vi "Main.vi"() -> ()   [LabVIEW 2013, in "Simple Sequence Editor.lvlib"]
uses:
  Simple Sequence Editor.lvlib
  Types/UI.PropertiesTypes.ctl
  Types/StateVariables.ctl
  Types/ChannelProperties.ctl
  <vilib>/Utility/miscctls.llb/LVBoundsTypeDef.ctl
panel:
  in  "Sequence":i32[](listbox)
  in  "View":T1=enum."Sequence Properties"
  in  "Abort Channel":string(combo)
  in  "Step Information Channel":string(combo)
  out "Graph":waveform(dbl)[](graph)
  out "Path":path
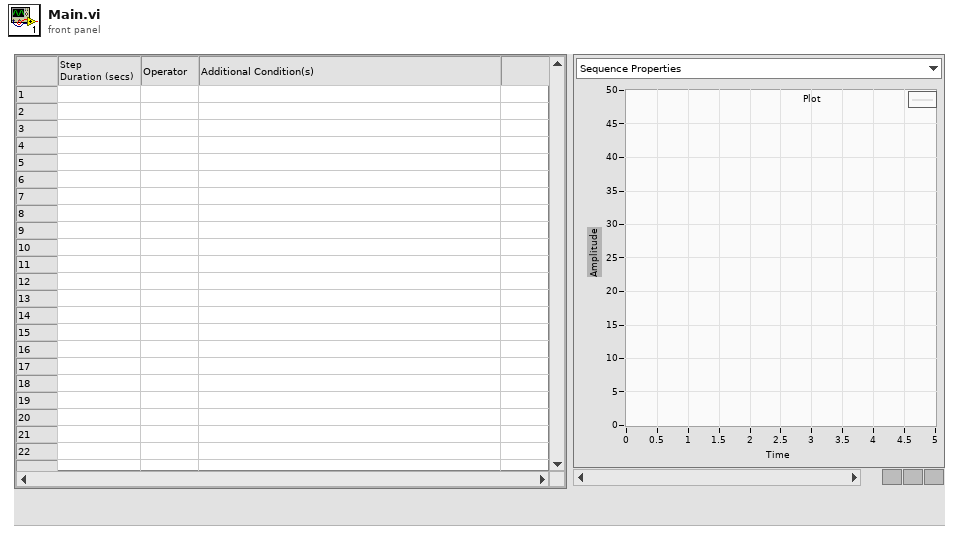
[diagram p1: front panel]
types:
  T1 = typedef "Simple Sequence Editor.lvlib/UI.PropertiesTypes.ctl" = enum8{"Step Properties", "Sequence Properties"}
  T2 = typedef "Simple Sequence Editor.lvlib/StateVariables.ctl" = cluster{"Aliases.All":T3[], "Aliases.Outputs":T3[], "UI.Sequence#ofColumns":i32, "SysDef.Path":path, "UI.SequenceRef":refnum<vi>, "UI.StepInformationRef":refnum<vi>, "UI.AbortRef":refnum<vi>, "UI.GraphRef":refnum<vi>, "UI.ViewRef":refnum<vi>}
  T3 = typedef "Simple Sequence Editor.lvlib/ChannelProperties.ctl" = cluster{"Name":string, "NodePath":string, "ScaleUnits":string}
  T4 = typedef "LVBoundsTypeDef.ctl" = cluster{"Width":u32, "Height":u32}
  T5 = enum16{"open", "replace", "create", "open or create", "replace or create", "replace or create with confirmation"}
  T6 = typedef "LVPoint32TypeDef.ctl" = cluster{"Horizontal":i32, "Vertical":i32}
  T7 = typedef "Simple Sequence Editor.lvlib/Compiled.RTSequenceProperties.ctl" = cluster{"Channels":T3[], "Steps":T8[]}
  T8 = typedef "Simple Sequence Editor.lvlib/Compiled.StepProperties.ctl" = cluster{"IOState":T9, "Condition":T12}
  T9 = typedef "Simple Sequence Editor.lvlib/Compiled.IOStateProperties.ctl" = cluster{"Duration":dbl, "Elements":T10[]}
  T10 = typedef "Simple Sequence Editor.lvlib/Compiled.StepElementProperties.ctl" = cluster{"Channel":T3, "Step":T11, "Parameters":dbl[]}
  T11 = typedef "Simple Sequence Editor.lvlib/StepTypes.ctl" = enum8{"Step", "iStep", "Ramp", "Unchanged", "Unknown"}
  T12 = typedef "Simple Sequence Editor.lvlib/Compiled.StepCondition.ctl" = cluster{"First Opreation":T13, "Expression":string}
  T13 = typedef "Simple Sequence Editor.lvlib/OperationTypes.ctl" = enum8{"None", "&&", "||"}
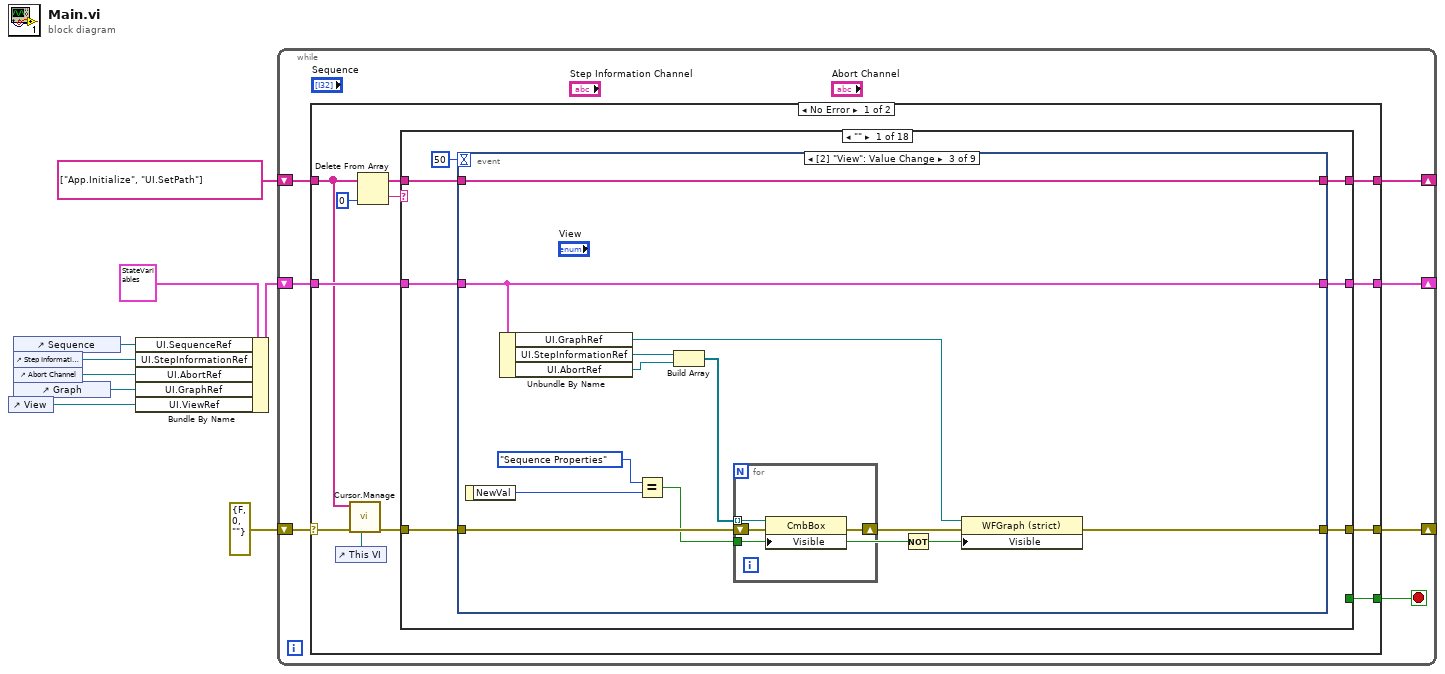
[diagram p0: block diagram]
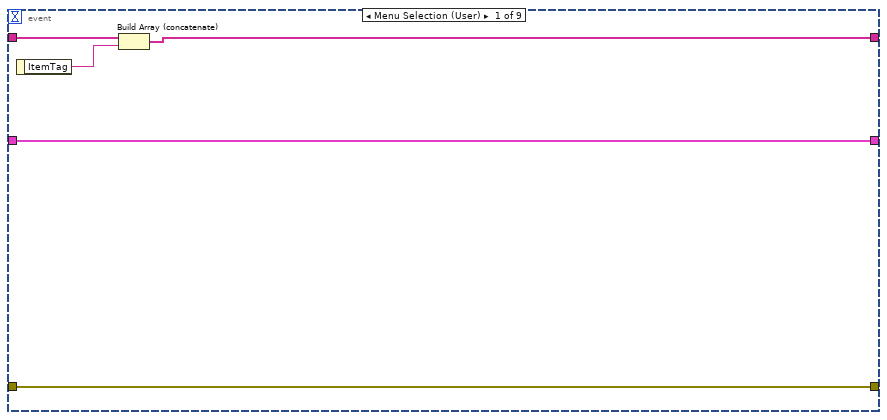
[diagram p2: hidden frame]
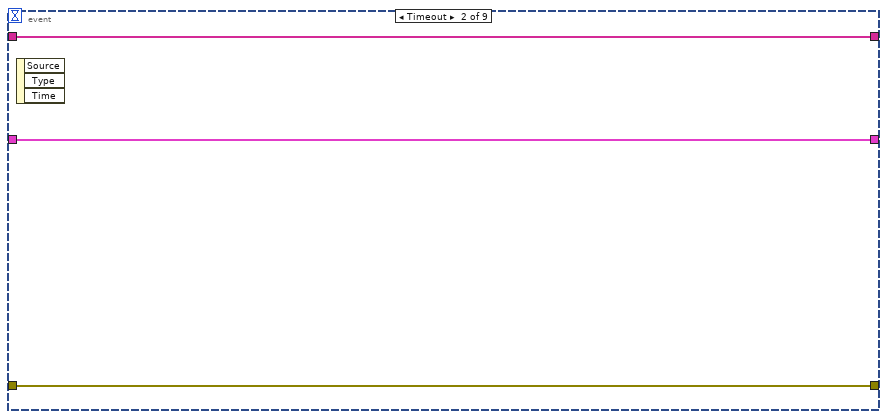
[diagram p3: hidden frame]
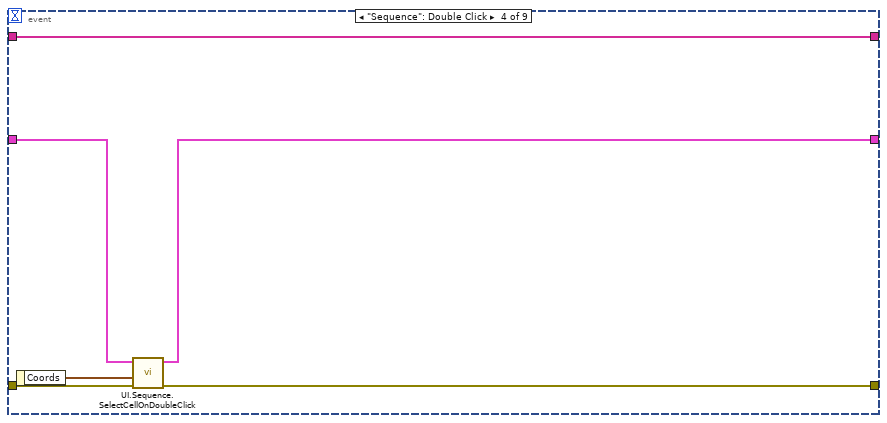
[diagram p4: hidden frame]
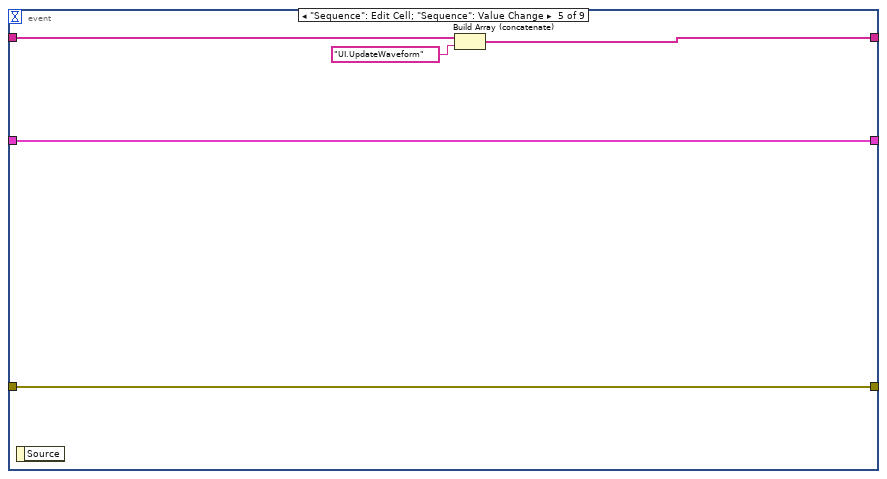
[diagram p5: hidden frame]
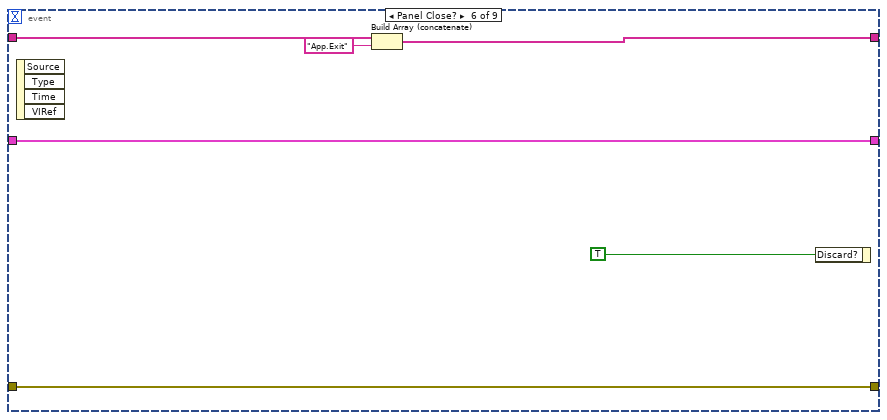
[diagram p6: hidden frame]
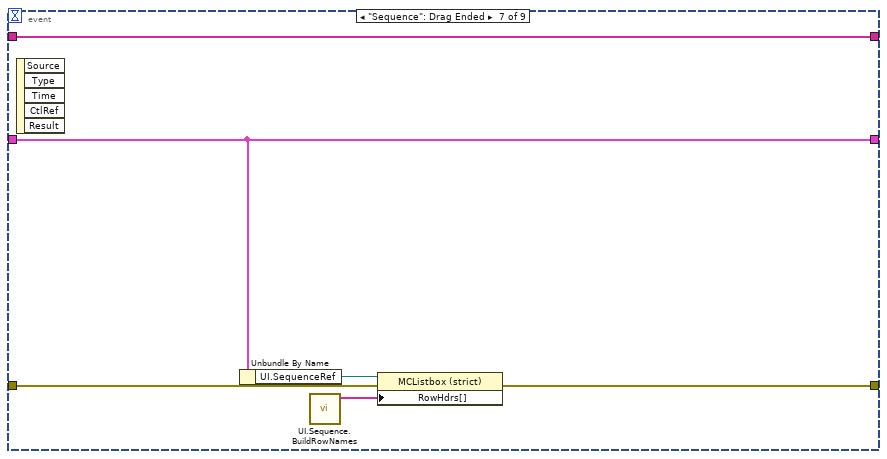
[diagram p7: hidden frame]
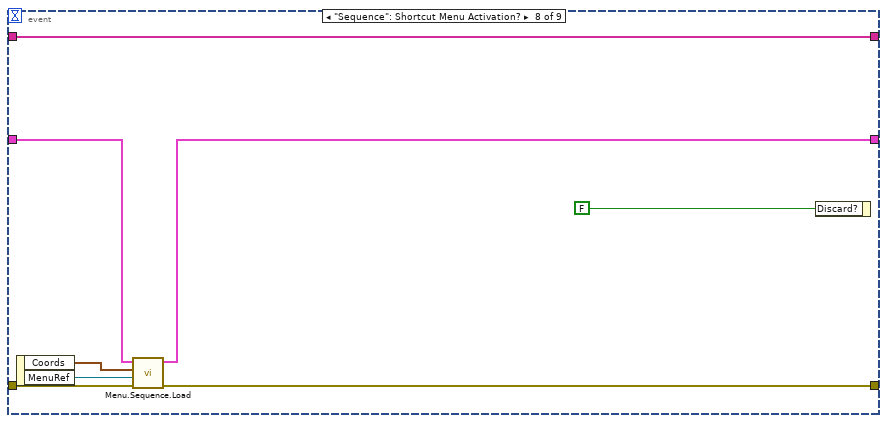
[diagram p8: hidden frame]
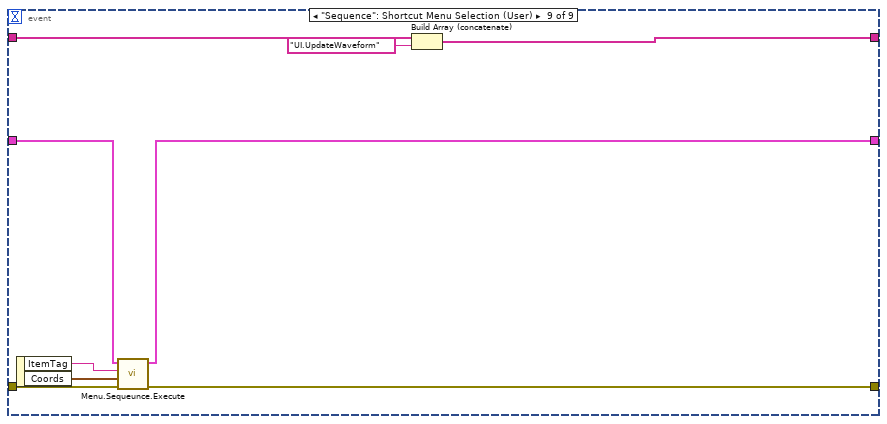
[diagram p9: hidden frame]
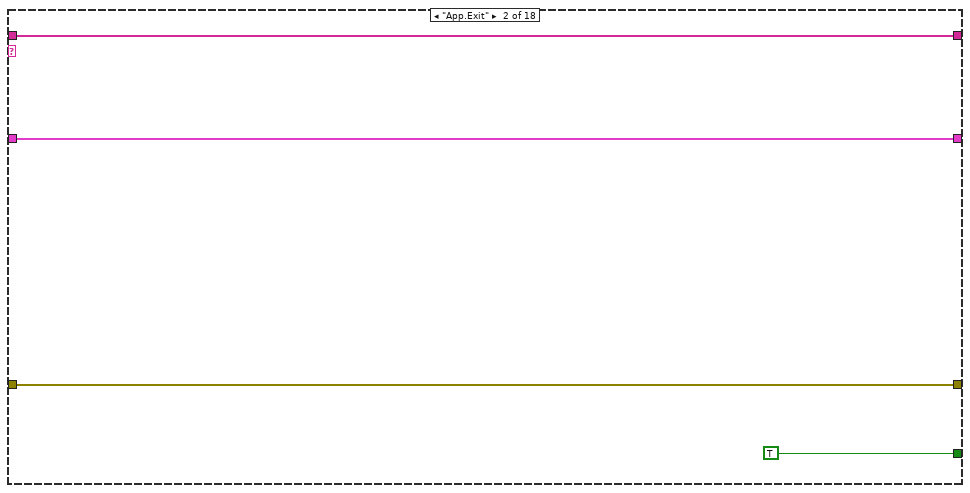
[diagram p10: hidden frame]
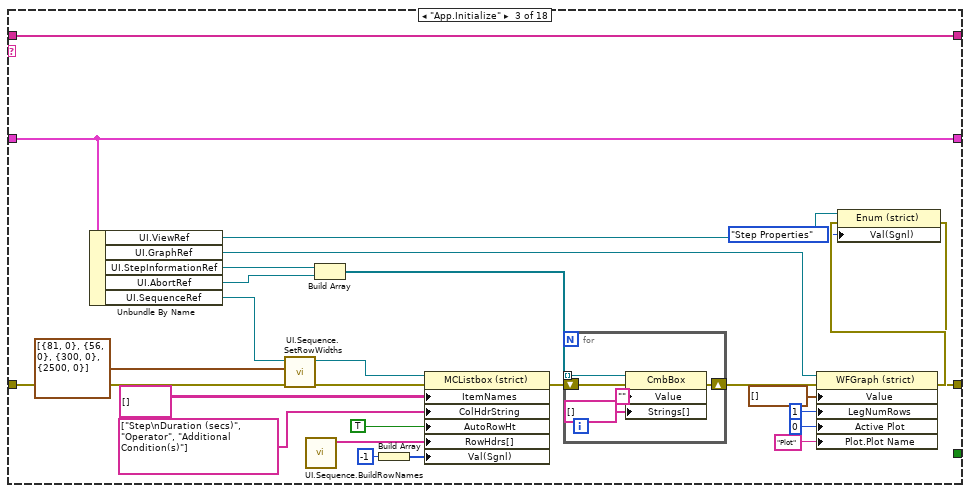
[diagram p11: hidden frame]
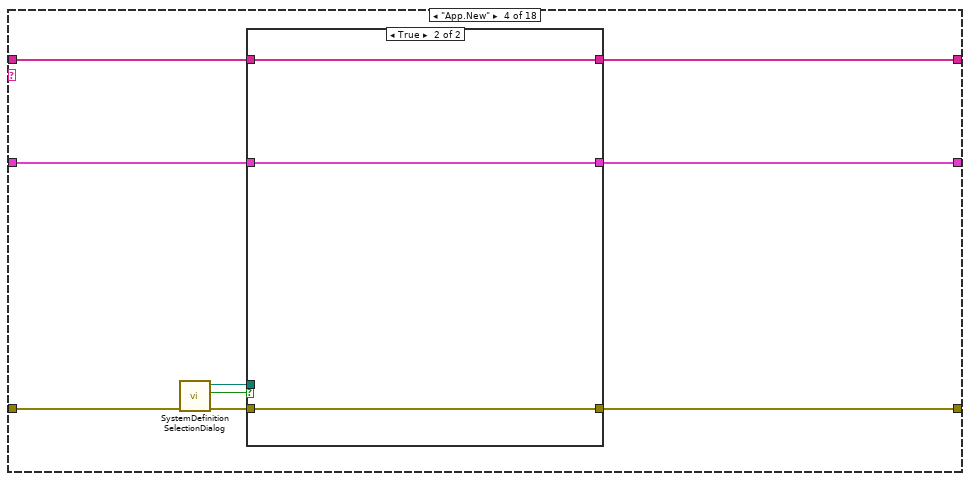
[diagram p12: hidden frame]
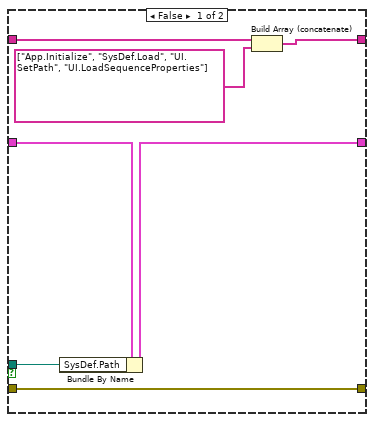
[diagram p13: hidden frame]
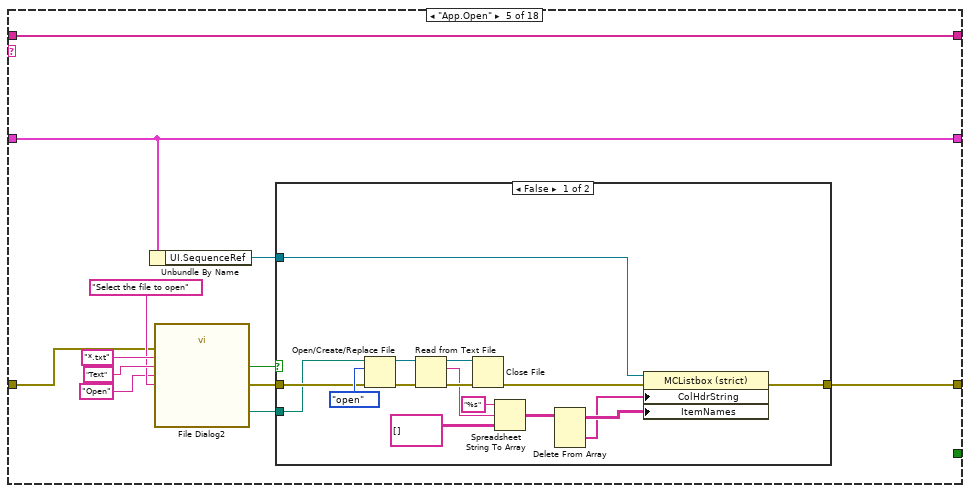
[diagram p14: hidden frame]
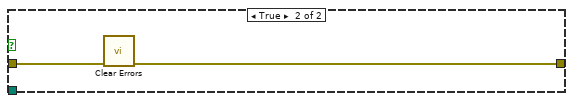
[diagram p15: hidden frame]
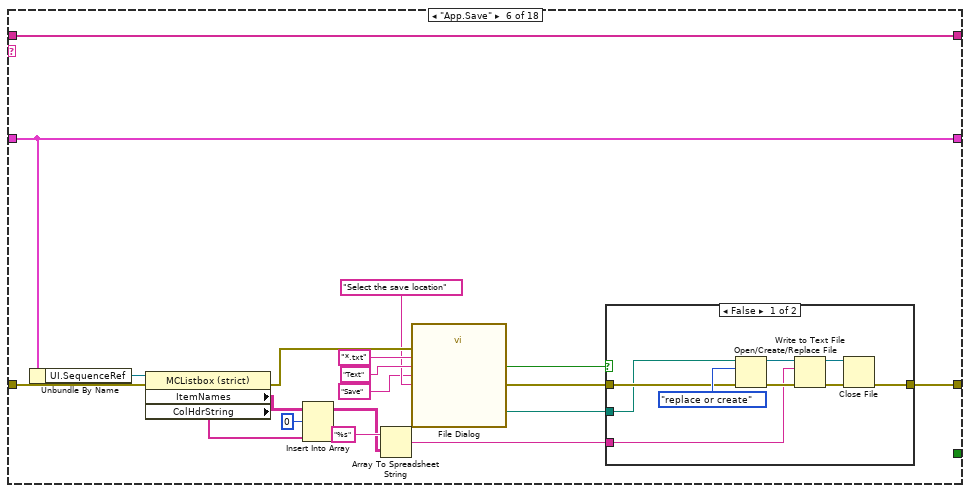
[diagram p16: hidden frame]
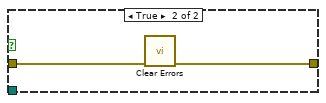
[diagram p17: hidden frame]
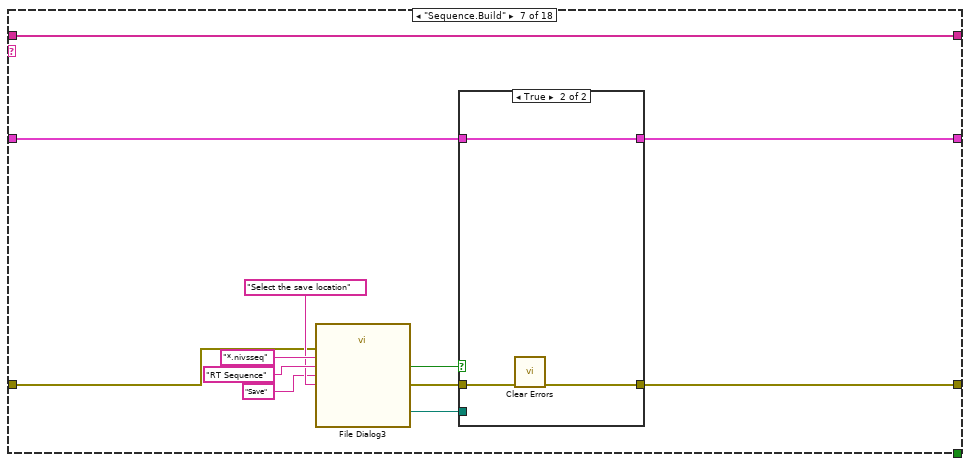
[diagram p18: hidden frame]
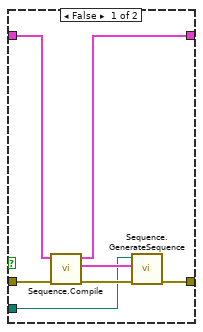
[diagram p19: hidden frame]
diagram:
  n1 = control-ref of="View"() -> (w1:refnum<vi>)
  n2 = control-ref of="Sequence"() -> (w5:refnum<vi>)
  n3 = control-ref of="Step Information Channel"() -> (w4:refnum<vi>)
  n4 = control-ref of="Abort Channel"() -> (w3:refnum<vi>)
  n5 = control-ref of="Graph"() -> (w2:refnum<vi>)
  n6 = Bundle By Name(cluster=T2 {"Aliases.All"=[], "Aliases.Outputs"=[], "UI.Sequence#ofColumns"=0, "SysDef.Path"=path "", "UI.SequenceRef"=refnum, "UI.StepInformationRef"=refnum, "UI.AbortRef"=refnum, "UI.GraphRef"=refnum, "UI.ViewRef"=refnum}, "UI.SequenceRef"=w5, "UI.StepInformationRef"=w4, "UI.AbortRef"=w3, "UI.GraphRef"=w2, "UI.ViewRef"=w1) -> (w6:T2)
  n7 = while {
    shift-right: [w15] -> _
    shift-left: string[] ["App.Initialize", "UI.SetPath"] -> [w16]
    shift-right: [w13] -> _
    shift-left: w6 -> [w14]
    shift-right: [w11] -> _
    shift-left: errorcluster {"status"=FALSE, "code"=0, "source"=""} ("error constant") -> [w12]
    stop <- w10 stop-if-true
    n8 = case shown="No Error" w12 {
      selector: w12 -> [w20 w326]
      tunnel: w16 -> [w21 w329]
      tunnel: [w27 w329] -> w15
      tunnel: w14 -> [w25 w328]
      tunnel: [w24 w328] -> w13
      tunnel: [w23 w325] -> w11
      tunnel: [w22 _] -> w10
      frame No Error {
        n9 = control-ref of="This VI"() -> (w17:refnum<vi>)
        n10 = call "Cursor.Manage.vi"("VI reference (current VI)"=w17, "error in (no error)"=w20, "Cmd list"=w21) -> ("error out"=w19:errorcluster)  [unwired: 8 in]
        n11 = Delete From Array(array=w21, index=0) -> (deleted portion=w28:string, array with subset deleted=w26:string[])  [unwired: 1 in]
        n12 = case shown="\"\"" w28 {
          tunnel: [w32 w104 w131 w137 w167 w204 w227 w240 w244 w250 w266 w267 w289 w294 w298 w312 w321 w324] -> w27
          tunnel: w26 -> [w31 w104 w131 w138 w167 w204 w227 w240 w244 w250 w266 w268 w290 w294 w298 w312 w321 w324]
          tunnel: w25 -> [w34 w103 w130 w141 w157 w203 w217 w239 w243 w249 w263 w271 w286 w291 w296 w307 w320 w323]
          tunnel: [w35 w103 w130 w139 w157 w203 w216 w239 w243 w249 w262 w269 w286 w291 w296 w308 w320 w323] -> w24
          tunnel: [w29 w102 w107 w142 w158 w199 w226 w238 w241 w247 w264 w272 w287 w292 w297 w309 w313 w322] -> w23
          tunnel: w19 -> [w30 w102 w125 w144 w159 w201 w221 w238 w242 w248 w259 w274 w287 w293 w297 w305 w314 w322]
          tunnel: [_ TRUE _ _ _ _ _ _ _ _ _ _ _ _ _ _ _ _] -> w22
          frame "" {
            n13 = event shown="[2] \"View\": Value Change" {
              selector: _ -> [_ _ _ _ _ _ _ _ _]
              dyn-events: _ -> [_ _ _ _ _ _ _ _ _]
              timeout: 50 -> [_ _ _ _ _ _ _ _ _]
              tunnel: [w37 w43 w56 w66 w68 w73 w83 w91 w93] -> w32
              tunnel: w31 -> [w39 w43 w56 w66 w71 w77 w83 w91 w100]
              tunnel: [w40 w42 w55 w61 w70 w76 w79 w87 w94] -> w35
              tunnel: w34 -> [w40 w42 w55 w62 w70 w76 w79 w84 w95]
              tunnel: [w38 w41 w47 w63 w69 w75 w80 w88 w96] -> w29
              tunnel: w30 -> [w38 w41 w51 w64 w69 w75 w81 w89 w97]
              event Menu Selection (User) {
                n14 = event-data() -> ("ItemTag"=w36:string)  [unwired: 1 in]
                n15 = Build Array (concatenate)(w39, w36) -> (w37:string[])
              }
              event Timeout {
                n16 = event-data() -> ()  [unwired: 1 in, 3 out]
              }
              event Value Change {
                n17 = event-data() -> ("NewVal"=w49:T1)  [unwired: 1 in]
                n18 = Unbundle By Name(w55) -> ("UI.GraphRef"=w46:refnum<vi>, "UI.StepInformationRef"=w54:refnum<vi>, "UI.AbortRef"=w53:refnum<vi>)
                n19 = Equal?(x=UI.PropertiesTypes."Sequence Properties" ("View"), y=w49) -> (x = y?=w45:bool)
                n20 = Build Array(w54, w53) -> (w52:refnum<vi>[])
                n21 = for {
                  tunnel: w52 -> [w60] mode=indexing
                  shift-right: [w58] -> w48
                  shift-left: w51 -> [w59]
                  tunnel: w45 -> [w57]
                  n22 = property class="CmbBox"(reference=w60, error in=w59, "Visible"=w57) -> (error out=w58:errorcluster)  [unwired: 1 out]
                }
                n23 = Not(x=w45) -> (.not. x?=w44:bool)
                n24 = property class="WFGraph (strict)"(reference=w46, error in=w48, "Visible"=w44) -> (error out=w47:errorcluster)  [unwired: 1 out]
              }
              event "Sequence": Double Click {
                n25 = event-data() -> ("Coords"=w65:T6)  [unwired: 1 in]
                n26 = call "UI.Sequence.SelectCellOnDoubleClick.vi"("error in (no error)"=w64, "Coords"=w65, "Cluster"=w62) -> ("error out"=w63:errorcluster, "Cluster out"=w61:T2)  [unwired: 7 in]
              }
              event "Sequence": Edit Cell; "Sequence": Value Change {
                n27 = event-data() -> ()  [unwired: 1 in, 1 out]
                n28 = Build Array (concatenate)(w71, "UI.UpdateWaveform" ("message")) -> (w68:string[])
              }
              event Panel Close? {
                n29 = event-data() -> ()  [unwired: 1 in, 4 out]
                n30 = Build Array (concatenate)(w77, "App.Exit") -> (w73:string[])
                n31 = event-data("Discard?"=TRUE) -> ()  [unwired: 1 in, 1 out]
              }
              event "Sequence": Drag Ended {
                n32 = event-data() -> ()  [unwired: 1 in, 5 out]
                n33 = Unbundle By Name(w79) -> ("UI.SequenceRef"=w78:refnum<vi>)
                n34 = call "UI.Sequence.BuildRowNames.vi"() -> ("Array"=w82:string[])  [unwired: 11 in]
                n35 = property class="MCListbox (strict)"(reference=w78, error in=w81, "RowHdrs[]"=w82) -> (error out=w80:errorcluster)  [unwired: 1 out]
              }
              event "Sequence": Shortcut Menu Activation? {
                n36 = event-data() -> ("Coords"=w85:T6, "MenuRef"=w86:refnum<k9>)  [unwired: 1 in]
                n37 = call "Menu.Sequence.Load.vi"("error in (no error)"=w89, "MenuRef"=w86, "Coords"=w85, "Cluster in"=w84) -> ("error out"=w88:errorcluster, "Cluster out"=w87:T2)  [unwired: 6 in]
                n38 = event-data("Discard?"=FALSE) -> ()  [unwired: 1 in, 1 out]
              }
              event "Sequence": Shortcut Menu Selection (User) {
                n39 = event-data() -> ("ItemTag"=w99:string, "Coords"=w98:T6)  [unwired: 1 in]
                n40 = call "Menu.Sequeunce.Execute.vi"("error in (no error)"=w97, "Coords"=w98, "ItemPath"=w99, "Cluster in"=w95) -> ("error out"=w96:errorcluster, "Cluster out"=w94:T2)  [unwired: 6 in]
                n41 = Build Array (concatenate)(w100, "UI.UpdateWaveform" ("message")) -> (w93:string[])
              }
            }
          }
          frame "App.Exit" {
          }
          frame "App.Initialize" {
            n42 = Unbundle By Name(w130) -> ("UI.ViewRef"=w109:refnum<vi>, "UI.GraphRef"=w115:refnum<vi>, "UI.StepInformationRef"=w117:refnum<vi>, "UI.AbortRef"=w118:refnum<vi>, "UI.SequenceRef"=w123:refnum<vi>)
            n43 = call "UI.Sequence.SetRowWidths.vi"("error in (no error)"=w125, "Array"=T4[] [{"Width"=81, "Height"=0}, {"Width"=56, "Height"=0}, {"Width"=300, "Height"=0}, {"Width"=2500, "Height"=0}], "UI.SequenceRef"=w123) -> ("error out"=w124:errorcluster, "UI.SequenceRef"=w122:refnum<vi>)  [unwired: 7 in]
            n44 = call "UI.Sequence.BuildRowNames.vi"() -> ("Array"=w121:string[])  [unwired: 11 in]
            n45 = Build Array(w117, w118) -> (w116:refnum<vi>[])
            n46 = Build Array(-1 ("Value")) -> (w119:i32[])
            n47 = property class="MCListbox (strict)"(reference=w122, error in=w124, "ItemNames"=string[][] [] ("Item Names"), "ColHdrString"=string[] ["Step\nDuration (secs)", "Operator", "Additional Condition(s)"] ("Column Header Strings[]"), "AutoRowHt"=TRUE ("Autosizing Row Height"), "RowHdrs[]"=w121, "Val(Sgnl)"=w119) -> (error out=w105:errorcluster)  [unwired: 1 out]
            n48 = for {
              tunnel: w116 -> [w135] mode=indexing
              shift-right: [w133] -> w114
              shift-left: w105 -> [w136]
              n49 = property class="CmbBox"(reference=w135, error in=w136, "Value"="", "Strings[]"=string[] [] ("Strings []")) -> (error out=w133:errorcluster)  [unwired: 1 out]
            }
            n50 = property class="WFGraph (strict)"(reference=w115, error in=w114, "Value"=waveform(dbl)[] [], "LegNumRows"=u32 1 ("Legend:Number of Rows"), "Active Plot"=u32 0, "Plot.Plot Name"="Plot") -> (error out=w108:errorcluster)  [unwired: 1 out]
            n51 = property class="Enum (strict)"(reference=w109, error in=w108, "Val(Sgnl)"=UI.PropertiesTypes."Step Properties" ("Value (Signaling)")) -> (error out=w107:errorcluster)  [unwired: 1 out]
          }
          frame "App.New" {
            n52 = call "SystemDefinitionSelectionDialog.vi"("error in (no error)"=w144) -> ("error out"=w145:errorcluster, "cancelled"=w143:bool, "selected path"=w140:path)  [unwired: 8 in]
            n53 = case shown="True" w143 {
              tunnel: w145 -> [w152 w154]
              tunnel: [w152 w154] -> w142
              tunnel: w141 -> [w151 w155]
              tunnel: [w150 w155] -> w139
              tunnel: w140 -> [w149 _]
              tunnel: [w148 w153] -> w137
              tunnel: w138 -> [w146 w153]
              frame False {
                n54 = Bundle By Name(cluster=w151, "SysDef.Path"=w149) -> (w150:T2)
                n55 = Build Array (concatenate)(w146, string[] ["App.Initialize", "SysDef.Load", "UI.SetPath", "UI.LoadSequenceProperties"]) -> (w148:string[])
              }
              frame True {
              }
            }
          }
          frame "App.Open" {
            n56 = Unbundle By Name(w157) -> ("UI.SequenceRef"=w156:refnum<vi>)
            n57 = call "File Dialog2"("prompt"="Select the file to open", "button label"="Open", "error in"=w159, "pattern (all files)"="*.txt", "pattern label"="Text") -> ("selected path"=w162:path, "cancelled"=w161:bool, "error out"=w166:errorcluster)  [unwired: 7 in, 1 out]
            n58 = case shown="False" w161 {
              tunnel: [w175 w184] -> w158
              tunnel: w166 -> [w178 w185]
              tunnel: w162 -> [w177 _]
              tunnel: w156 -> [w174 _]
              frame False {
                n59 = Open/Create/Replace File(file path (use dialog)=w177, error in=w178, operation (0:open)=T5."open") -> (refnum out=w180:refnum<file>, error out=w183:errorcluster)  [unwired: 3 in, 1 out]
                n60 = Read from Text File(file (use dialog)=w180, error in=w183) -> (refnum out=w181:refnum<file>, text=w173:string, error out=w182:errorcluster)  [unwired: 2 in, 1 out]
                n61 = Close File(refnum=w181, error in=w182) -> (error out=w176:errorcluster)  [unwired: 1 out]
                n62 = Spreadsheet String To Array(format string="%s", spreadsheet string=w173, array type (2D Dbl)=string[][] []) -> (array=w170:string[][])  [unwired: 1 in]
                n63 = Delete From Array(array=w170) -> (deleted portion=w168:string[], array with subset deleted=w169:string[][])  [unwired: 3 in]
                n64 = property class="MCListbox (strict)"(reference=w174, error in=w176, "ColHdrString"=w168, "ItemNames"=w169) -> (error out=w175:errorcluster)  [unwired: 1 out]
              }
              frame True {
                n65 = call <vilib>:"Clear Errors.vi"("error in (no error)"=w185) -> ("error out"=w184:errorcluster)  [unwired: 6 in]
              }
            }
          }
          frame "App.Save" {
            n66 = Unbundle By Name(w203) -> ("UI.SequenceRef"=w202:refnum<vi>)
            n67 = property class="MCListbox (strict)"(reference=w202, error in=w201) -> (error out=w197:errorcluster, "ItemNames"=w188:string[][], "ColHdrString"=w186:string[])  [unwired: 1 out]
            n68 = Insert Into Array(array=w188, index (row)=0, new element=w186) -> (w189:string[][])  [unwired: 1 in]
            n69 = Array To Spreadsheet String(array=w189, 3:"%s" ("format string")) -> (spreadsheet string=w198:string)  [unwired: 1 in]
            n70 = call "File Dialog"("prompt"="Select the save location", "button label"="Save", "error in"=w197, "pattern (all files)"="*.txt", "pattern label"="Text") -> ("selected path"=w192:path, "cancelled"=w191:bool, "error out"=w196:errorcluster)  [unwired: 7 in, 1 out]
            n71 = case shown="False" w191 {
              tunnel: [w209 w214] -> w199
              tunnel: w198 -> [w208 _]
              tunnel: w196 -> [w206 w215]
              tunnel: w192 -> [w205 _]
              frame False {
                n72 = Open/Create/Replace File(file path (use dialog)=w205, error in=w206, operation (0:open)=T5."replace or create") -> (refnum out=w210:refnum<file>, error out=w213:errorcluster)  [unwired: 3 in, 1 out]
                n73 = Write to Text File(file (use dialog)=w210, text=w208, error in=w213) -> (refnum out=w211:refnum<file>, error out=w212:errorcluster)  [unwired: 1 in, 1 out]
                n74 = Close File(refnum=w211, error in=w212) -> (error out=w209:errorcluster)  [unwired: 1 out]
              }
              frame True {
                n75 = call <vilib>:"Clear Errors.vi"("error in (no error)"=w215) -> ("error out"=w214:errorcluster)  [unwired: 6 in]
              }
            }
          }
          frame "Sequence.Build" {
            n76 = call "File Dialog3"("prompt"="Select the save location", "button label"="Save", "error in"=w221, "pattern (all files)"="*.nivsseq", "pattern label"="RT Sequence") -> ("selected path"=w220:path, "cancelled"=w219:bool, "error out"=w218:errorcluster)  [unwired: 7 in, 1 out]
            n77 = case shown="True" w219 {
              tunnel: w217 -> [w234 w236]
              tunnel: [w231 w235] -> w226
              tunnel: w218 -> [w230 w237]
              tunnel: w220 -> [w229 _]
              tunnel: [w228 w236] -> w216
              frame False {
                n78 = call "Sequence.Compile.vi"("error in (no error)"=w230, "input cluster"=w234) -> ("error out"=w232:errorcluster, 2:"output cluster"=w233:T7, 3:"output cluster"=w228:T2)  [unwired: 7 in]
                n79 = call "Sequence.GenerateSequence.vi"("error in (no error)"=w232, "output cluster"=w233, "Path"=w229) -> ("error out"=w231:errorcluster)  [unwired: 8 in]
              }
              frame True {
                n80 = call <vilib>:"Clear Errors.vi"("error in (no error)"=w237) -> ("error out"=w235:errorcluster)  [unwired: 6 in]
              }
            }
          }
          frame "Sequence.Validate" {
          }
          frame "Sequence.Preview" {
            n81 = call "Sequence.Preview.vi"("error in (no error)"=w242, "input cluster"=w243) -> ("error out"=w241:errorcluster)  [unwired: 9 in]
          }
          frame "SysDef.Edit" {
            n82 = Unbundle By Name(w249) -> ("SysDef.Path"=w246:path)
            n83 = Empty String/Path?(string/path=w246) -> (empty?=w245:bool)
            n84 = case shown="True" w245 {
              tunnel: w248 -> [w257 w258]
              tunnel: [w256 w258] -> w247
              tunnel: w246 -> [w255 _]
              frame False {
                # "Launch VeriStand and open systemdefinition"
                n85 = Path To String(path=w255) -> (string=w254:string)
                n86 = Concatenate Strings("explorer " ("string"), w254) -> (w252:string)
                n87 = call <vilib>:"System Exec.vi"("run minimized? (F)"=TRUE, "error in (no error)"=w257, "command line"=w252) -> ("error out"=w256:errorcluster)  [unwired: 5 in, 3 out]
              }
              frame True {
              }
            }
          }
          frame "SysDef.Load" {
            n88 = Unbundle By Name(w263) -> ("SysDef.Path"=w265:path)
            n89 = call "LoadSystemDefinition.vi"("error in (no error)"=w259, "SysDef.Path"=w265) -> ("error out"=w264:errorcluster, "Aliases.Outputs"=w260:T3[], "Aliases.All"=w261:T3[])  [unwired: 7 in]
            n90 = Bundle By Name(cluster=w263, "Aliases.All"=w261, "Aliases.Outputs"=w260) -> (w262:T2)
          }
          frame "SysDef.New" {
            n91 = call "SystemDefinitionSelectionDialog.vi"("error in (no error)"=w274) -> ("error out"=w275:errorcluster, "cancelled"=w273:bool, "selected path"=w270:path)  [unwired: 8 in]
            n92 = case shown="False" w273 {
              tunnel: w275 -> [w282 w284]
              tunnel: [w282 w284] -> w272
              tunnel: w271 -> [w281 w285]
              tunnel: [w280 w285] -> w269
              tunnel: w270 -> [w279 _]
              tunnel: [w278 w283] -> w267
              tunnel: w268 -> [w276 w283]
              frame False {
                n93 = Bundle By Name(cluster=w281, "SysDef.Path"=w279) -> (w280:T2)
                n94 = Build Array (concatenate)(w276, string[] ["SysDef.Load", "UI.SetPath", "UI.LoadSequenceProperties"]) -> (w278:string[])
              }
              frame True {
              }
            }
          }
          frame "SysDef.Refresh" {
            n95 = Build Array (concatenate)(w290, string[] ["SysDef.Load", "UI.SetPath", "UI.LoadSequenceProperties"]) -> (w289:string[])
          }
          frame "Steps.GenerateMultiple" {
            n96 = call "Dialog.MassStepGeneration.vi"("error in (no error)"=w293, "Cluster"=w291) -> ("error out"=w292:errorcluster)  [unwired: 9 in]
          }
          frame "UI.SetPath" {
            n97 = Unbundle By Name(w296) -> ("SysDef.Path"=→"Path":path)
          }
          frame "UI.UpdateWaveform" {
            n98 = Unbundle By Name(w307) -> ("UI.SequenceRef"=w306:refnum<vi>)
            n99 = property class="MCListbox (strict)"(reference=w306, error in=w305) -> (error out=w304:errorcluster, "Value"=w300:i32[])  [unwired: 1 out]
            n100 = Index Array(array=w300) -> (element=w299:i32)  [unwired: 1 in]
            n101 = Array Size(array=w300) -> (size(s)=w301:i32)
            n102 = Bundle By Name(cluster=cluster{"Start Index":i32, "Length":i32} {"Start Index"=0, "Length"=-1} ("Rows"), "Start Index"=w299, "Length"=w301) -> (w302:cluster{"Start Index":i32, "Length":i32})
            n103 = control-ref of="Graph"() -> (w311:refnum<vi>)
            n104 = call "Sequence.BuildPreviewWaveform.vi"("WaveformGraph in"=w311, "error in (no error)"=w304, "Rows"=w302, "input cluster"=w307) -> ("error out"=w309:errorcluster, "Wavefrom"=→"Graph":waveform(dbl)[], "input cluster out"=w308:T2)  [unwired: 5 in]
          }
          frame "UI.LoadSequenceProperties" {
            n105 = Unbundle By Name(w320) -> ("UI.StepInformationRef"=w316:refnum<vi>, "UI.AbortRef"=w318:refnum<vi>, "Aliases.All"=w319:T3[])
            n106 = call "Channel.BuildMenuName.vi"("Aliases"=w319) -> ("Aliases Array"=w315:string[])  [unwired: 10 in]
            n107 = property class="CmbBox"(reference=w318, error in=w314, "Strings[]"=w315) -> (error out=w317:errorcluster)  [unwired: 1 out]
            n108 = property class="CmbBox"(reference=w316, error in=w317, "Strings[]"=w315) -> (error out=w313:errorcluster)  [unwired: 1 out]
          }
          frame Default {
          }
        }
      }
      frame Error {
        n109 = call <vilib>:"Simple Error Handler.vi"("error in (no error)"=w326) -> ("error out"=w327:errorcluster)  [unwired: 4 in, 4 out]
        n110 = call <vilib>:"Clear Errors.vi"("error in (no error)"=w327) -> ("error out"=w325:errorcluster)  [unwired: 6 in]
      }
    }
  }
